vi "End Unit of Work.vi"(8 "error in (no error)":errorcluster, 11 "Entity Manager in":refnum<class "Entity Manager.lvclass">) -> (0 "error out":errorcluster, 3 "Entity Manager out":refnum<class "Entity Manager.lvclass">)   [LabVIEW 2020, in "Conditu2.lvlib" / "Entity Manager.lvclass"]
uses:
  Entity Manager.lvclass
  Entity Manager.lvclass/Entity Manager.ctl
  Unit Of Work Session/Unit Of Work Session.lvclass
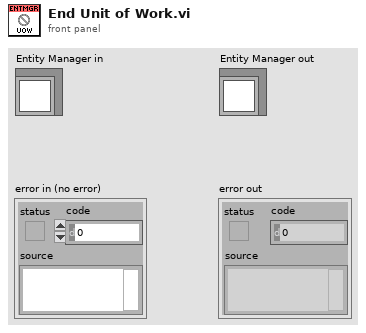
[diagram p1: front panel]
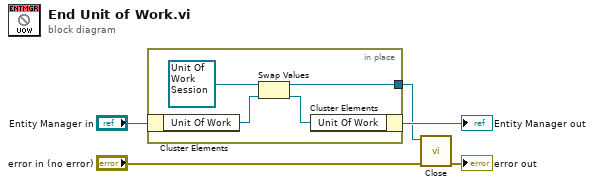
[diagram p0: block diagram]
diagram:
  n1 = in-place {
    in-place-border: [w6] -> w3
    n2 = in-place-cluster #1("Entity Manager in") -> ("Unit Of Work"=w8:refnum<class "Unit Of Work Session.lvclass">)
    n3 = Swap Values(12:refnum<class "Unit Of Work Session.lvclass"> refnum ("Unit Of Work"), 14:w8) -> (1:w6:refnum<class "Unit Of Work Session.lvclass">, 3:w7:refnum<class "Unit Of Work Session.lvclass">)  [unwired: 1 in]
    n4 = in-place-cluster #1("Unit Of Work"=w7) -> (→"Entity Manager out":refnum<class "Entity Manager.lvclass">)
  }
  n5 = call "Close.vi"("error in (no error)"="error in (no error)", "Unit Of Work in"=w3) -> ("error out"=→"error out":errorcluster)  [unwired: 9 in]
